vi "ImportProject.vi"(8 "error in (no error)":errorcluster, 10 "XML File Path":path, 11 "ProjectManager in":refnum<class "XML Project.lvclass">) -> (0 "error out":errorcluster, 2 "value":refnum<class "BrowerComponent.lvclass">, 3 "ProjectManager out":refnum<class "XML Project.lvclass">)   [LabVIEW 2015, in "XML Project.lvclass"]
uses:
  XML Project.lvclass
  Brower Console/Models/BrowerComponent/BrowerComponent/BrowerComponent.lvclass
  <vilib>/Utility/xml.llb/Read From XML File(string).vi
panel:
  out "SymbolIndex":i32
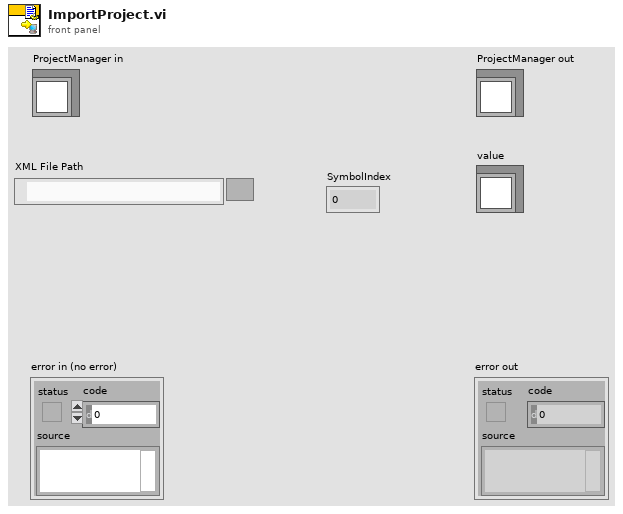
[diagram p1: front panel]
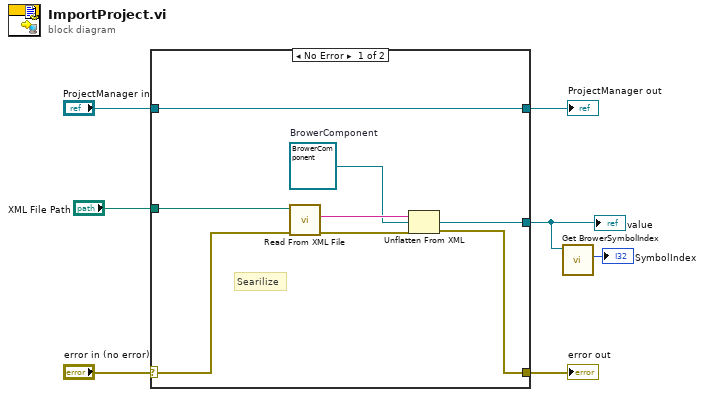
[diagram p0: block diagram]
diagram:
  n1 = case shown="No Error" "error in (no error)" {
    selector: "error in (no error)" -> [w13 w17]
    tunnel: [w9 w17] -> w6
    tunnel: [w15 w16] -> w4
    tunnel: "ProjectManager in" -> [w15 w16]
    tunnel: "XML File Path" -> [w14 _]
    tunnel: [w8 _] -> w2
    frame No Error {
      w10 = refnum<class "BrowerComponent.lvclass"> refnum  # BrowerComponent
      # "Searilize"
      n2 = call-poly <vilib>:"Read From XML File.vi"("error in (no error)"=w13, "XML File Path"=w14) -> ("error out"=w12:errorcluster, "XML Elements"=w11:string)  [unwired: 7 in, 1 out]
      n3 = Unflatten From XML(xml string=w11, type=w10, error in (no error)=w12) -> (value=w8:refnum<class "BrowerComponent.lvclass">, error out=w9:errorcluster)
    }
    frame Error {
    }
  }
  "error out" <- w6
  "ProjectManager out" <- w4
  "value" <- w2
  n4 = call "Get BrowerSymbolIndex.vi"("BrowerComponent in"=w2) -> ("SymbolIndex"=→"SymbolIndex":i32)  [unwired: 8 in, 2 out]
